vi "H5Sget_select_hyper_blocklist.vi"(6 "error in (no error)":errorcluster, 7 "Numpoints (All)":i32=-1, 8 "Start (0)":u64, 9 "HDF5 Space Ref":T1) -> (0 "error out":errorcluster, 2 "Hyperslab Blocks":cluster{"Start":u64[], "Opposite":u64[]}[](array[cluster]), 3 "HDF5 Ref out":T1)   [LabVIEW 2017]
doc: "Gets the list of hyperslab blocks currently selected."
uses:
  <vilib>/UPVI/lvhdf5/library.llb/HDF5 Ref.ctl
  <vilib>/UPVI/lvhdf5/hdf5.dll
panel:
  # "LVHDF5 Toolkit\nCopyright (c) 2005-2013 by Jason D. Sommerville\nCopyright (c) 2014 by UPVI, LLC.\n\nThis use and distribution of this file is governed by the terms found in \nLICENSE.txt distributed with this toolkit and installed at\n <user.lib>\\_lvhdf5\\LICENSE.txt"
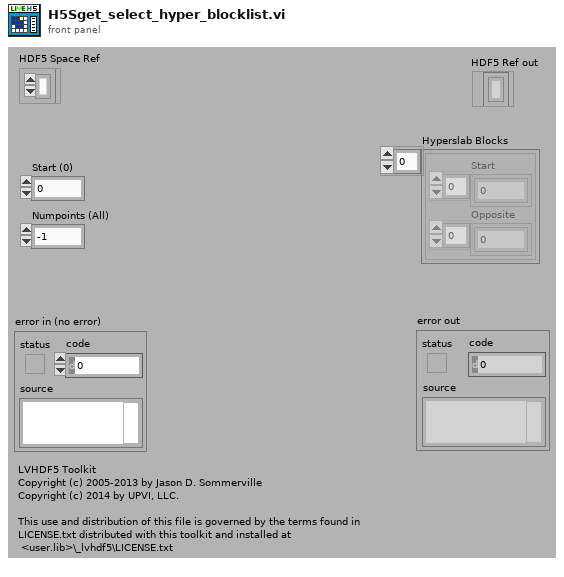
[diagram p1: front panel]
types:
  T1 = typedef "HDF5 Ref.ctl" = refnum<k1>
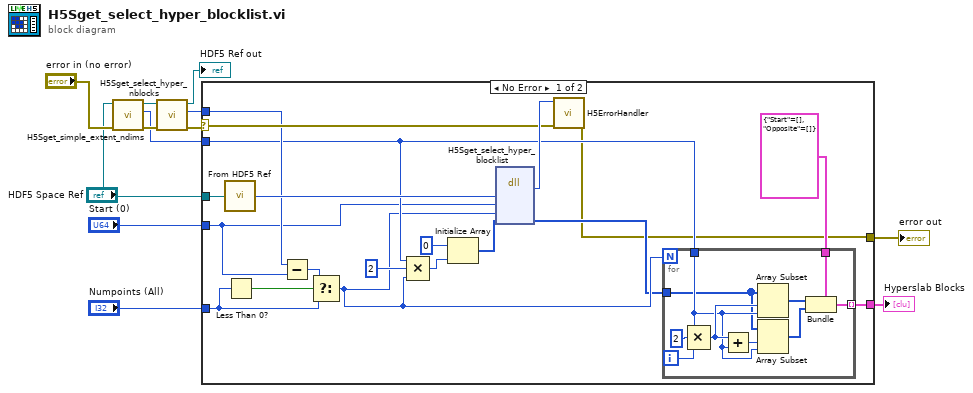
[diagram p0: block diagram]
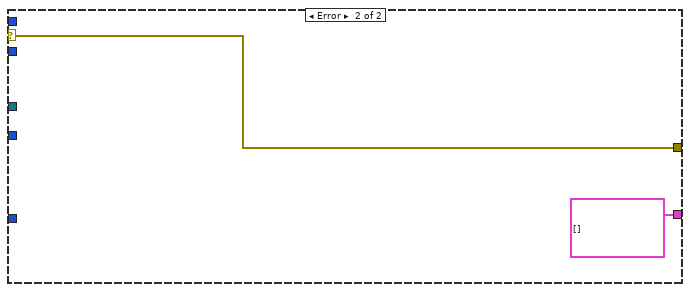
[diagram p2: hidden frame]
diagram:
  n1 = call <vilib>:"H5Sget_simple_extent_ndims.vi"("error in (no error)"="error in (no error)", "HDF5 Space Ref"="HDF5 Space Ref") -> ("error out"=w5:errorcluster, "Rank"=w2:i32, "HDF5 Ref out"=w3:T1)  [unwired: 5 in]
  n2 = call <vilib>:"H5Sget_select_hyper_nblocks.vi"("error in (no error)"=w5, "HDF5 Space Ref"=w3) -> ("error out"=w9:errorcluster, "Count"=w7:i64, "HDF5 Ref out"=→"HDF5 Ref out":T1)  [unwired: 5 in]
  n3 = case shown="No Error" w9 {
    selector: w9 -> [w28 w43]
    tunnel: [w13 w43] -> w12
    tunnel: "HDF5 Space Ref" -> [w31 _]
    tunnel: "Start (0)" -> [w15 _]
    tunnel: "Numpoints (All)" -> [w25 _]
    tunnel: w7 -> [w26 _]
    tunnel: w2 -> [w18 _]
    tunnel: [w21 cluster{"Start":i32[], "Opposite":i32[]}[] []] -> w1
    frame No Error {
      n4 = call <vilib>:"From HDF5 Ref.vi"("HDF5 Ref"=w31) -> ("I32"=w30:i32)
      n5 = Less Than 0?(x=w25) -> (x < 0?=w27:bool)
      n6 = Subtract(x=w26, y=w15) -> (x-y=w24:u64)
      n7 = Select(t=w24, s=w27, f=w25) -> (s? t:f=w16:u64)
      n8 = Compound Arithmetic op=MULTIPLY(w18, 2 ("y"), w16) -> (w17:u64)
      n9 = Initialize Array(u64 0, w17) -> (w20:u64[])
      n10 = dll-call lib="C:/Program Files/National Instruments/LabVIEW 2017/vi.lib/UPVI/lvhdf5/hdf5.dll" fn="H5Sget_select_hyper_blocklist"("space_id"=w30, "startpoint"=w15, "numpoints"=w16, "pointlist"=w20) -> ("return type"=w29:i32, "pointlist"=w14:u64[])  [unwired: 6 in, 2 out]
      n11 = call <vilib>:"H5ErrorHandler.vi"("error in (no error)"=w28, "herr_t"=w29) -> ("error out"=w13:errorcluster)  [unwired: 3 in, 4 out]
      n12 = for {
        N: w16 -> [_]
        tunnel: w14 -> [w32]
        tunnel: cluster{"Start":u64[], "Opposite":u64[]} {"Start"=[], "Opposite"=[]} ("cluster") -> [w39]
        tunnel: [w38] -> w21 mode=indexing
        tunnel: w18 -> [w34]
        i -> [w37]
        n13 = Compound Arithmetic op=MULTIPLY(w34, 2 ("y"), w37) -> (w35:i32)
        n14 = Add(x=w35, y=w34) -> (x+y=w36:i32)
        n15 = Array Subset(array=w32, index=w35, length=w34) -> (w40:u64[])
        n16 = Array Subset(array=w32, index=w36, length=w34) -> (w33:u64[])
        n17 = Bundle(cluster=w39, "Start"=w40, "Opposite"=w33) -> (w38:cluster{"Start":u64[], "Opposite":u64[]})
      }
    }
    frame Error {
    }
  }
  "error out" <- w12
  "Hyperslab Blocks" <- w1
